vi "Argument to Large String.vi"(11 "Arguments":string) -> (0 "error out":errorcluster, 3 "String":string)   [LabVIEW 2020, in "CSMScript-Engine(Lite).lvlib"]
uses:
  CSMScript-Engine(Lite).lvlib
  b50c31bd-cb45-49b6-b3a2-cde9c36a776d.vi
  <userlib>/_NEVSTOP/Communicable State Machine(CSM)/AdvanceAPI/CSM - Keywords.vi
  <userlib>/_NEVSTOP/Communicable State Machine(CSM)/addons/MassData-Parameter/_support/FGV-MassData(lvlibp).vi
  <userlib>/_NEVSTOP/Communicable State Machine(CSM)/_Shared/CSM Shared.lvlib
  <userlib>/_NEVSTOP/Communicable State Machine(CSM)/Communicable State Machine.lvlib
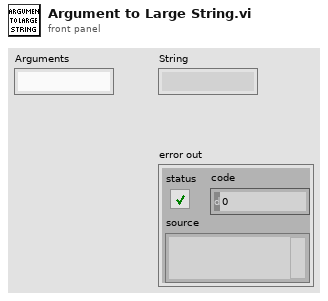
[diagram p1: front panel]
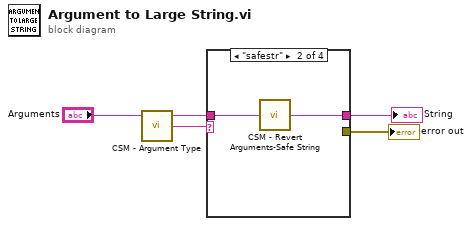
[diagram p0: block diagram]
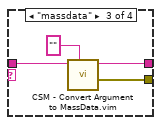
[diagram p3: hidden frame]
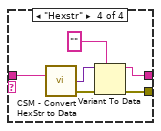
[diagram p4: hidden frame]
diagram:
  n1 = call <userlib>:"CSM - Argument Type.vi"("Arguments"="Arguments") -> ("Argument Type"=w5:string, "Arguments (Dup)"=w4:string)  [unwired: 3 in]
  n2 = case shown="\"safestr\"" w5 {
    tunnel: [_ w7 w10 w12] -> w2
    tunnel: w4 -> [_ w6 w11 w16]
    tunnel: [_ _ w8 w15] -> w1
    frame Default {
    }
    frame "safestr" {
      n3 = call <userlib>:"CSM - Revert Arguments-Safe String.vi"("Safe Argument String"=w6) -> ("Origin Argument String"=w7:string)  [unwired: 8 in]
    }
    frame "massdata" {
      n4 = call "CSM - Convert Argument to MassData.vim"("Type"="" ("Init State(\"Macro: Initialize\")"), "MassData Argument"=w11) -> ("error out"=w8:errorcluster, "Data"=w10:string)  [unwired: 6 in]
    }
    frame "Hexstr" {
      n5 = call <userlib>:"CSM - Convert HexStr to Data.vi"("HEX String"=w16) -> ("Variant"=w14:variant, "error out"=w17:errorcluster)  [unwired: 7 in]
      n6 = Variant To Data(error in=w17, type="", Variant=w14) -> (data=w12:string, error out=w15:errorcluster)
    }
  }
  "String" <- w2
  "error out" <- w1
